vi "HDF5_Write_TC_Record.vi"(8 "error in":errorcluster, 10 "TCData":T1, 11 "TC_Refs":T2 {"TC13_Tamb_Inter" format="%.0x"; "TC12_Gen_Exhaust" format="%.0x"; "TC11_HVAC_Cond_Out" format="%.0x"; "TC10_HVAC_Cond_In" format="%.0x"; "TC9_LP2_Lo" format="%.0x"; "TC8_LP2_LoMid" format="%.0x"; "TC7_LP2_Mid" format="%.0x"; "TC6_LP2_MidHi" format="%.0x"; "TC5_LP2_Hi" format="%.0x"; "TC4_LP1_Lo" format="%.0x"; "TC3_LP1_LoMid" format="%.0x"; "TC2_LP1_Mid" format="%.0x"; "TC1_LP1_MidHi" format="%.0x"; "TC0_LP1_Hi" format="%.0x"; "TimeString_dset" format="%.0x"; "TimeStamp_dset" format="%.0x"; "Group_ref" format="%.0x"}) -> (0 "error out":errorcluster, 2 "date/time string":string, 3 "current time":timestamp)   [LabVIEW 2018]
doc: "Write a single Tone<x> record with timestamp:\nTone1\n Beac - cluster\n BeacZoom - 1024 element Double array (waveform) \n Cal - cluster\n CalZoom - 1024 element Double array (waveform)"
uses:
  TC_Tone_refs.ctl
  <vilib>/addons/h5labview2/base/hid_t.ctl
  TC_Data_Structure.ctl
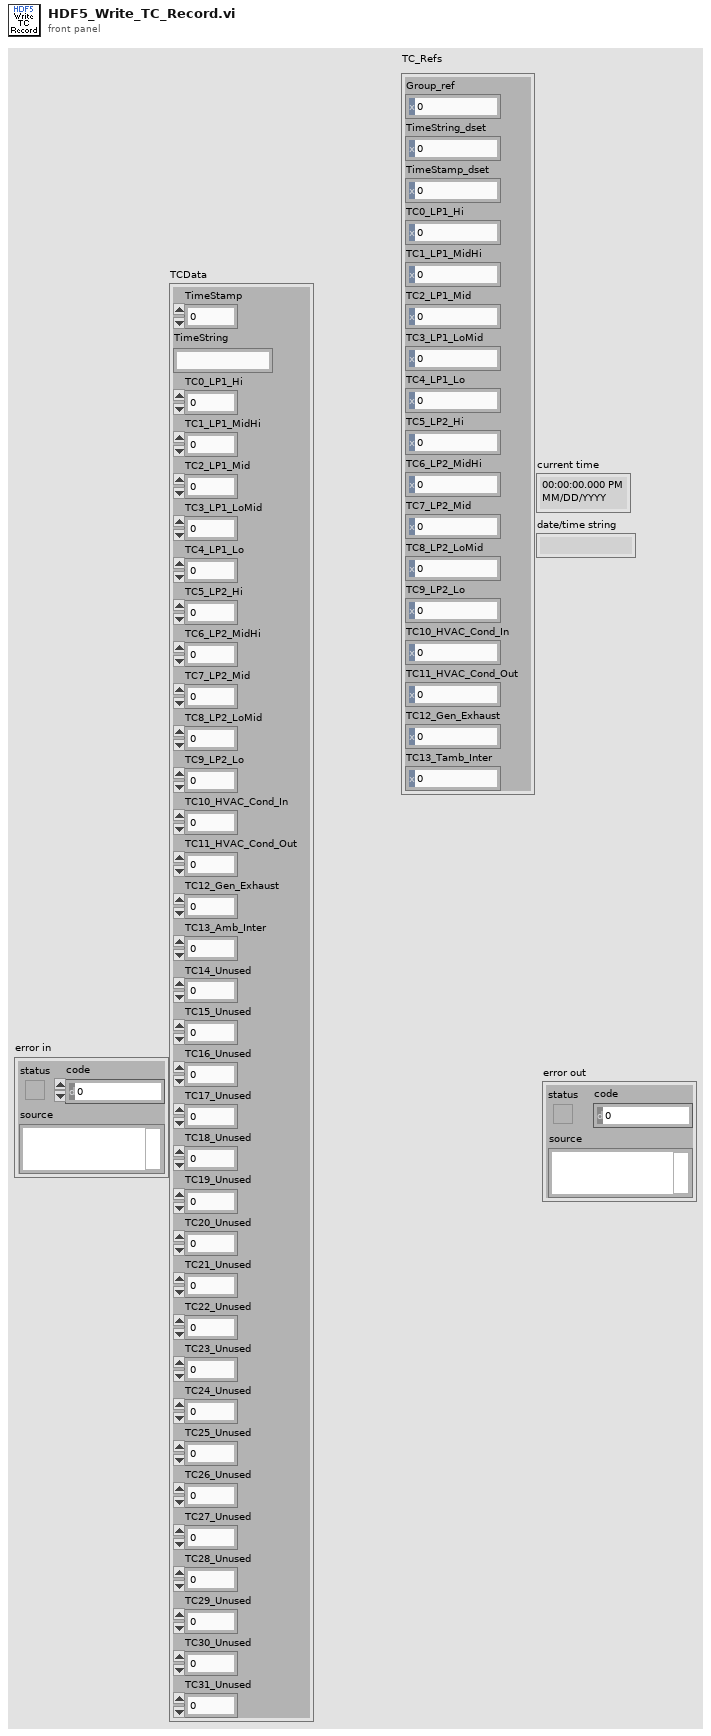
[diagram p1: front panel]
types:
  T1 = typedef "TC_Data_Structure.ctl" = cluster{"TimeStamp":dbl, "TimeString":string, "TC0_LP1_Hi":dbl, "TC1_LP1_MidHi":dbl, "TC2_LP1_Mid":dbl, "TC3_LP1_LoMid":dbl, "TC4_LP1_Lo":dbl, "TC5_LP2_Hi":dbl, "TC6_LP2_MidHi":dbl, "TC7_LP2_Mid":dbl, "TC8_LP2_LoMid":dbl, "TC9_LP2_Lo":dbl, "TC10_HVAC_Cond_In":dbl, "TC11_HVAC_Cond_Out":dbl, "TC12_Gen_Exhaust":dbl, "TC13_Amb_Inter":dbl, "TC14_Unused":dbl, "TC15_Unused":dbl, "TC16_Unused":dbl, "TC17_Unused":dbl, "TC18_Unused":dbl, "TC19_Unused":dbl, "TC20_Unused":dbl, "TC21_Unused":dbl, "TC22_Unused":dbl, "TC23_Unused":dbl, "TC24_Unused":dbl, "TC25_Unused":dbl, "TC26_Unused":dbl, "TC27_Unused":dbl, "TC28_Unused":dbl, "TC29_Unused":dbl, "TC30_Unused":dbl, "TC31_Unused":dbl}
  T2 = typedef "TC_Tone_refs.ctl" = cluster{"Group_ref":T3, "TimeString_dset":T3, "TimeStamp_dset":T3, "TC0_LP1_Hi":T3, "TC1_LP1_MidHi":T3, "TC2_LP1_Mid":T3, "TC3_LP1_LoMid":T3, "TC4_LP1_Lo":T3, "TC5_LP2_Hi":T3, "TC6_LP2_MidHi":T3, "TC7_LP2_Mid":T3, "TC8_LP2_LoMid":T3, "TC9_LP2_Lo":T3, "TC10_HVAC_Cond_In":T3, "TC11_HVAC_Cond_Out":T3, "TC12_Gen_Exhaust":T3, "TC13_Tamb_Inter":T3}
  T3 = typedef "hid_t.ctl" = i32
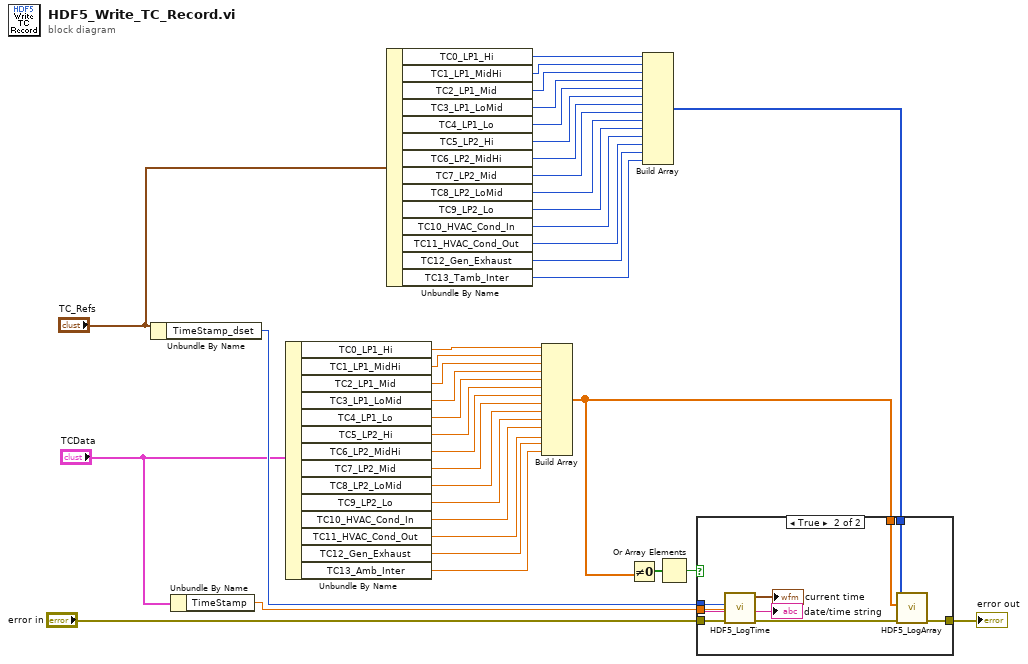
[diagram p0: block diagram]
diagram:
  n1 = Unbundle By Name("TC_Refs") -> ("TimeStamp_dset"=w36:T3)
  n2 = Unbundle By Name("TCData") -> ("TimeStamp"=w4:dbl)
  n3 = Unbundle By Name("TCData") -> ("TC0_LP1_Hi"=w6:dbl, "TC1_LP1_MidHi"=w7:dbl, "TC2_LP1_Mid"=w8:dbl, "TC3_LP1_LoMid"=w9:dbl, "TC4_LP1_Lo"=w10:dbl, "TC5_LP2_Hi"=w11:dbl, "TC6_LP2_MidHi"=w12:dbl, "TC7_LP2_Mid"=w13:dbl, "TC8_LP2_LoMid"=w14:dbl, "TC9_LP2_Lo"=w15:dbl, "TC10_HVAC_Cond_In"=w16:dbl, "TC11_HVAC_Cond_Out"=w17:dbl, "TC12_Gen_Exhaust"=w18:dbl, "TC13_Amb_Inter"=w19:dbl)
  n4 = Unbundle By Name("TC_Refs") -> ("TC0_LP1_Hi"=w34:T3, "TC1_LP1_MidHi"=w33:T3, "TC2_LP1_Mid"=w32:T3, "TC3_LP1_LoMid"=w31:T3, "TC4_LP1_Lo"=w30:T3, "TC5_LP2_Hi"=w29:T3, "TC6_LP2_MidHi"=w28:T3, "TC7_LP2_Mid"=w27:T3, "TC8_LP2_LoMid"=w26:T3, "TC9_LP2_Lo"=w25:T3, "TC10_HVAC_Cond_In"=w24:T3, "TC11_HVAC_Cond_Out"=w23:T3, "TC12_Gen_Exhaust"=w22:T3, "TC13_Tamb_Inter"=w21:T3)
  n5 = Build Array(w6, w7, w8, w9, w10, w11, w12, w13, w14, w15, w16, w17, w18, w19) -> (w2:dbl[])
  n6 = Not Equal To 0?(x=w2) -> (x != 0?=w3:bool[])
  n7 = Build Array(w34, w33, w32, w31, w30, w29, w28, w27, w26, w25, w24, w23, w22, w21) -> (w20:T3[])
  n8 = Or Array Elements(Boolean array=w3) -> (logical OR=w1:bool)
  n9 = case shown="True" w1 {
    tunnel: [w39 w48] -> w38
    tunnel: "error in" -> [w39 w47]
    tunnel: w36 -> [_ w46]
    tunnel: w20 -> [_ w44]
    tunnel: w2 -> [_ w43]
    tunnel: w4 -> [_ w40]
    frame False {
      # "Don't log if all values are zero."
    }
    frame True {
      n10 = call "HDF5_LogTime.vi"("error in (no error)"=w47, "Timestamp"=w40, "TimeStamp_dset"=w46) -> ("error out"=w45:errorcluster, "date/time string"=→"date/time string":string, "current time"=→"current time":timestamp)  [unwired: 6 in]
      n11 = call "HDF5_LogArray.vi"("error in (no error)"=w45, "array of Data"=w43, "array of Refs"=w44) -> ("error out"=w48:errorcluster)  [unwired: 8 in]
    }
  }
  "error out" <- w38
